vi "Write Standard.vi"(8 "error in (no error)":errorcluster, 10 "Standard":string, 11 "IMD_ACP in":refnum<class "IMD_ACP.lvclass">) -> (0 "error out":errorcluster, 3 "IMD_ACP out":refnum<class "IMD_ACP.lvclass">)   [LabVIEW 2018, in "SeqAuto Evaluations.lvlib" / "IMD_ACP.lvclass"]
uses:
  IMD_ACP.lvclass
  IMD_ACP.lvclass/IMD_ACP.ctl
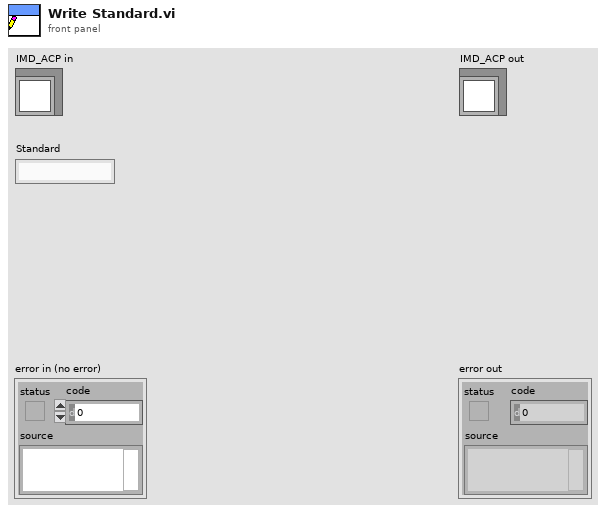
[diagram p1: front panel]
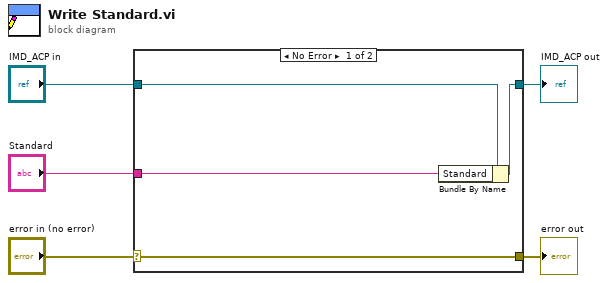
[diagram p0: block diagram]
diagram:
  n1 = case shown="No Error" "error in (no error)" {
    selector: "error in (no error)" -> [w9 w10]
    tunnel: [w9 w10] -> w4
    tunnel: [w7 w11] -> w2
    tunnel: "IMD_ACP in" -> [w8 w11]
    tunnel: "Standard" -> [w6 _]
    frame No Error {
      n2 = Bundle By Name(cluster=w8, "Standard"=w6) -> (w7:refnum<class "IMD_ACP.lvclass">)
    }
    frame Error {
    }
  }
  "error out" <- w4
  "IMD_ACP out" <- w2
